vi "pia datos.vi"() -> ()   [LabVIEW 2020]
uses:
  <vilib>/Instr/_visa.llb/VISA Configure Serial Port (Instr).vi
panel:
  out "Waveform Chart":i32(graph)
  out "POSICION ACTUAL DE BRAZO":i16(knob) scale=-1023.0..1023.0
  out "TRAMA":string
  in  "stop":bool
  in  "Seleccion de puerto":refnum<visa-resource-name>
  out "ERROR":i16(knob) scale=-400.0..400.0
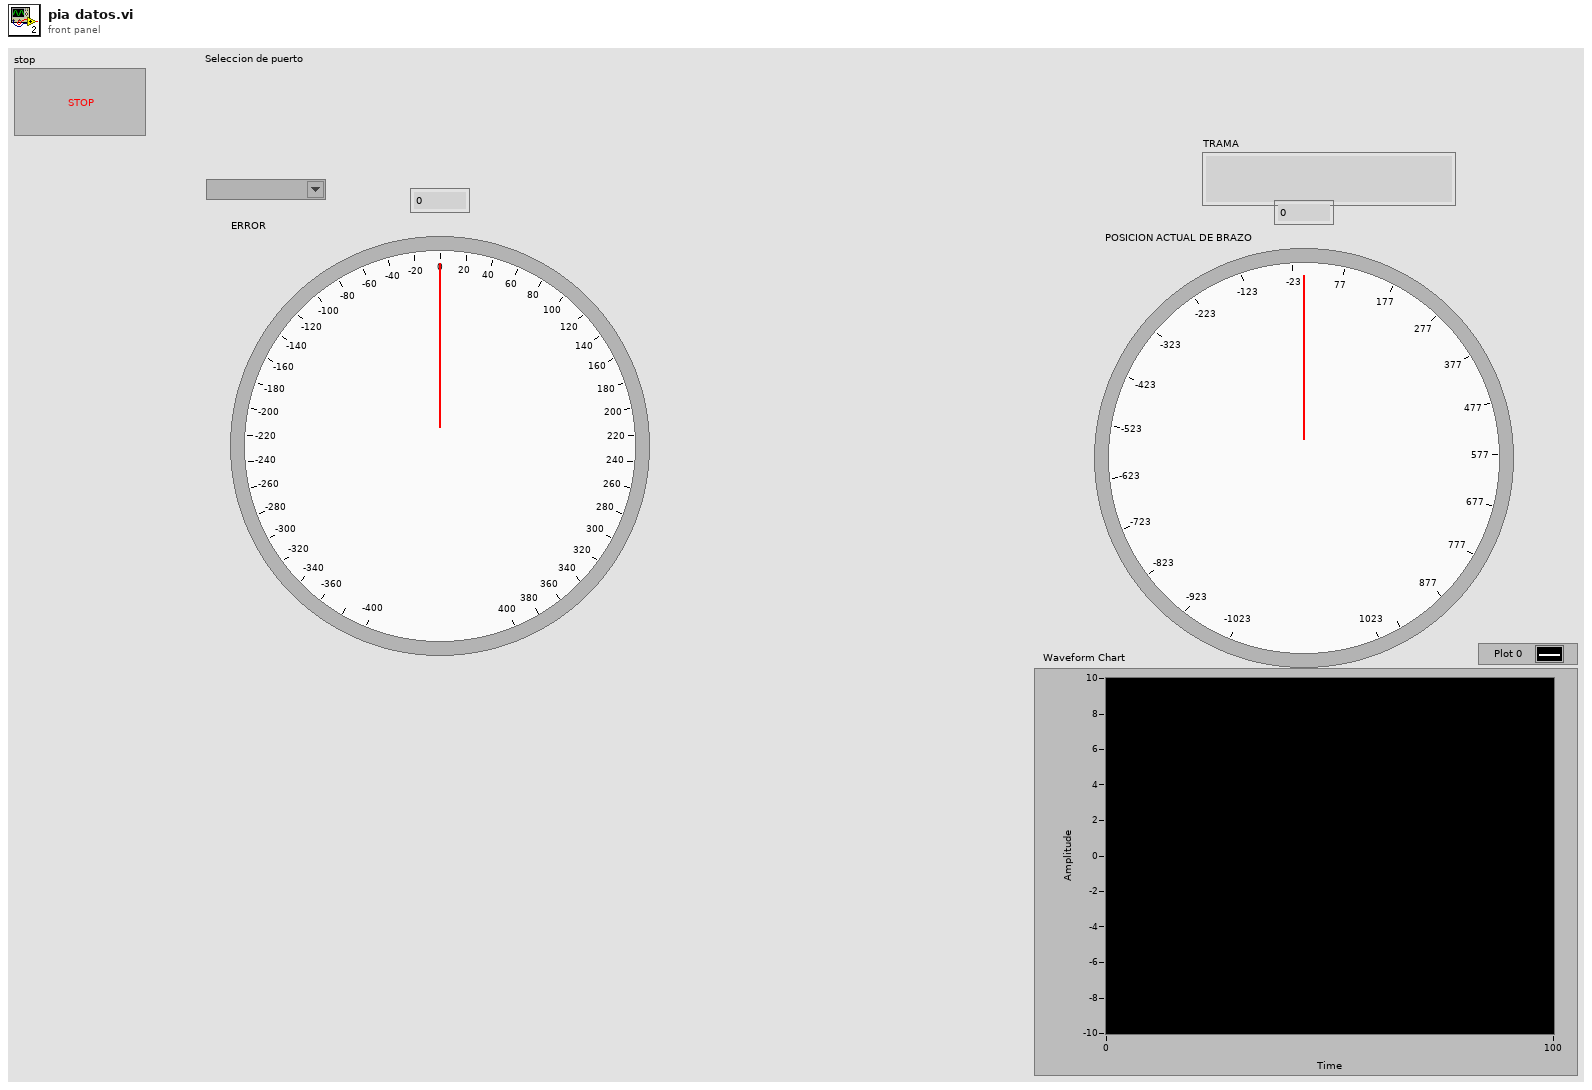
[diagram p1: front panel]
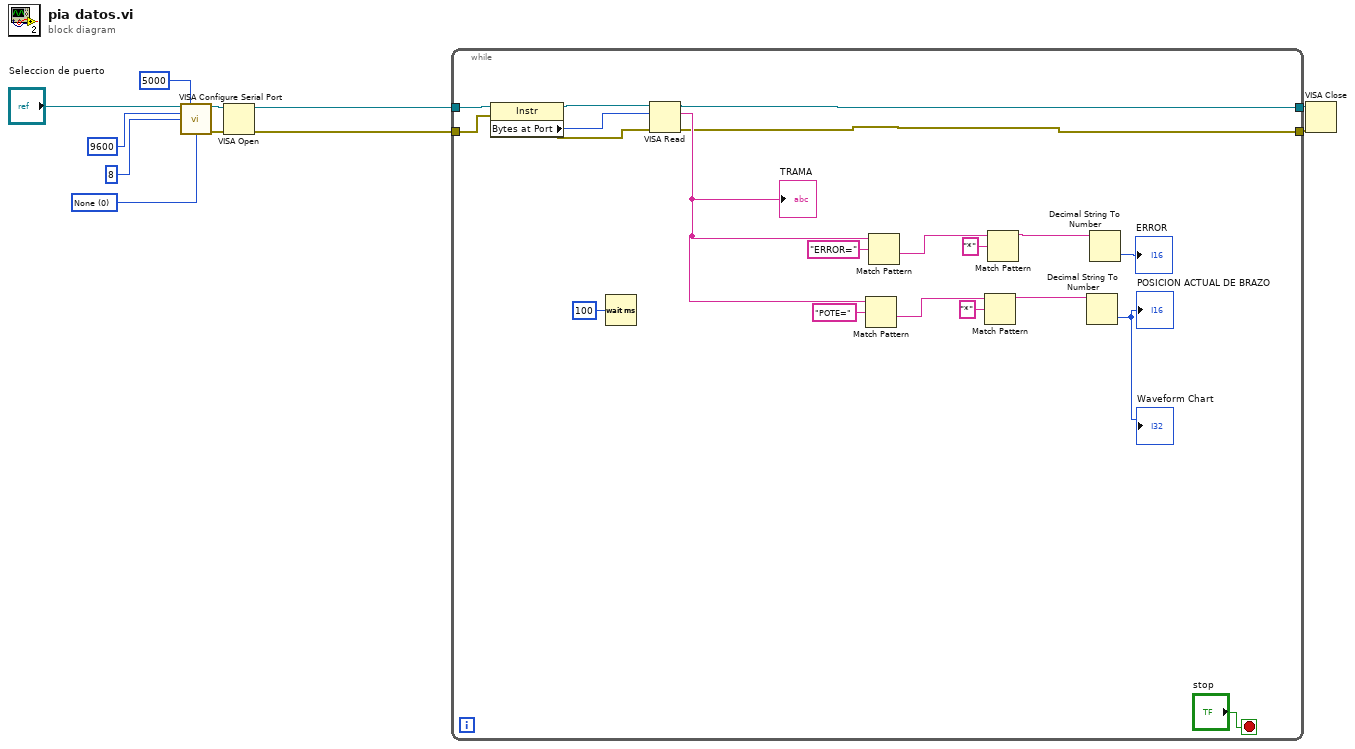
[diagram p0: block diagram]
diagram:
  w8 = u16 0 items=["None", "XON/XOFF", "RTS/CTS", "XON/XOFF & RTS/CTS", "DTR/DSR", "XON/XOFF & DTR/DSR"] ("flow control (0:none)")
  n1 = call-poly "VISA Configure Serial Port"("VISA resource name"="Seleccion de puerto", "timeout (10sec)"=u32 5000, "baud rate (9600)"=u32 9600, "data bits (8)"=u16 8, "flow control (0:none)"=w8) -> ("VISA resource name out"=w6:refnum<visa-resource-name>, "error out"=w5:errorcluster)  [unwired: 9 in]
  n2 = VISA Open(error in (no error)=w5, VISA resource name=w6) -> (VISA resource name=w2:refnum<visa-resource-name>, error out=w1:errorcluster)  [unwired: 3 in]
  n3 = while {
    tunnel: w2 -> [w29]
    tunnel: [w14] -> w4
    tunnel: w1 -> [w28]
    tunnel: [w13] -> w3
    stop <- "stop" stop-if-true
    n4 = property class="Instr"(reference=w29, error in=w28) -> (reference out=w16:refnum<visa-resource-name>, error out=w17:errorcluster, "Bytes at Port"=w18:u32)
    n5 = Wait (ms)(milliseconds to wait=u32 100) -> ()  [unwired: 1 out]
    n6 = VISA Read(VISA resource name=w16, byte count=w18, error in (no error)=w17) -> (VISA resource name out=w14:refnum<visa-resource-name>, read buffer=w19:string, error out=w13:errorcluster)  [unwired: 1 out]
    "TRAMA" <- w19
    n7 = Match Pattern(string=w19, regular expression="POTE=") -> (after substring=w21:string)  [unwired: 1 in, 3 out]
    n8 = Match Pattern(string=w19, regular expression="ERROR=") -> (after substring=w26:string)  [unwired: 1 in, 3 out]
    n9 = Match Pattern(string=w21, regular expression="*") -> (before substring=w15:string)  [unwired: 1 in, 3 out]
    n10 = Match Pattern(string=w26, regular expression="*") -> (before substring=w23:string)  [unwired: 1 in, 3 out]
    n11 = Decimal String To Number(string=w15) -> (number=→"POSICION ACTUAL DE BRAZO" →"Waveform Chart":i32)  [unwired: 2 in, 1 out]
    n12 = Decimal String To Number(string=w23) -> (number=→"ERROR":i32)  [unwired: 2 in, 1 out]
  }
  n13 = VISA Close(VISA resource name=w4, error in (no error)=w3) -> ()  [unwired: 1 out]
